vi "SQL_Template_selectidbyname.vi"(11 "模板名称":string) -> (0 "error out":errorcluster, 3 "tempNo":string)   [LabVIEW 2014]
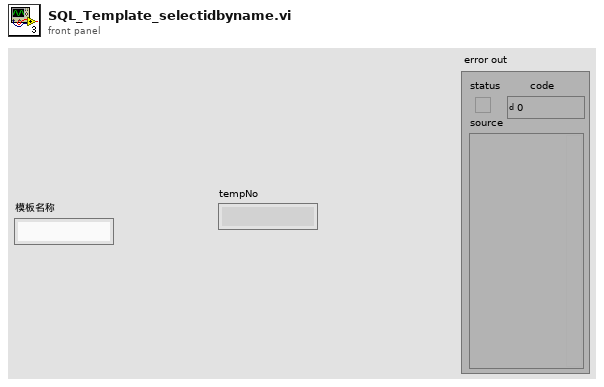
[diagram p1: front panel]
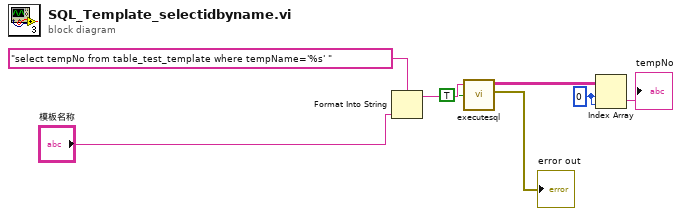
[diagram p0: block diagram]
diagram:
  w3 = 0 ("索引 (行)")
  n1 = Format Into String(format string="select tempNo from table_test_template where tempName='%s' ", "模板名称") -> (resulting string=w6:string)  [unwired: 2 in, 1 out]
  n2 = call "executesql.vi"("Return Data (T)"=TRUE, "Command Text"=w6) -> ("error out"=→"error out":errorcluster, "Data"=w4:string[][])  [unwired: 5 in]
  n3 = Index Array(array=w4, index (row)=w3, index (col)=w3) -> (element=→"tempNo":string)
